vi "Flatten to protobuf.vi"(8 "error in (no error)":errorcluster, 10 "Data":T1) -> (0 "error out":errorcluster, 2 "Buffer":u8[](array[numeric]) format="%.0x")   [LabVIEW 2020, in "PB Msg Template.lvlib"]
uses:
  PB Msg Template.lvlib
  Data.ctl
  LV-Proto/Wire Encode Tag.vi
  LV-Proto/Wire Encode Varint I32.vi
  LV-Proto/LV-Proto.lvlib
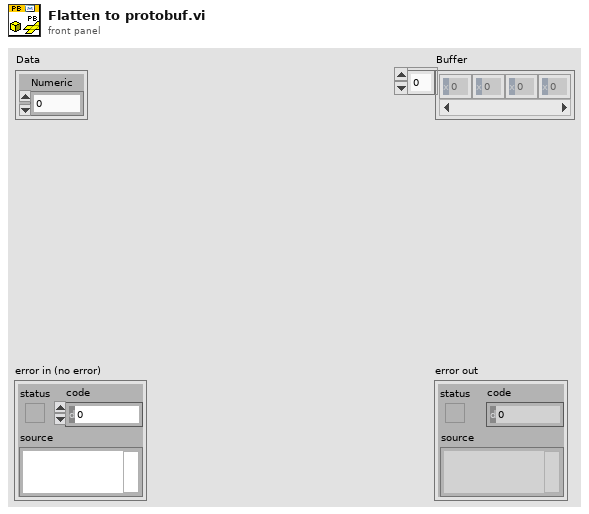
[diagram p1: front panel]
types:
  T1 = typedef "PB Msg Template.lvlib/Data.ctl" = cluster{"Numeric":dbl}
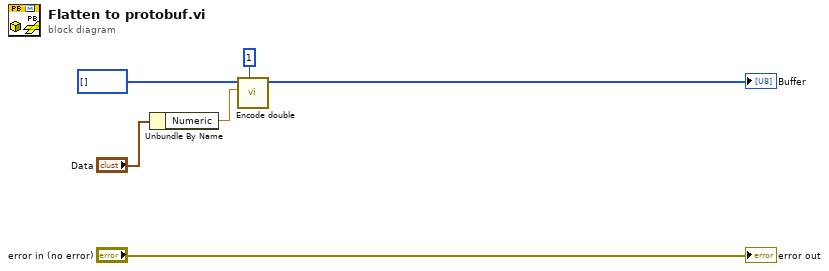
[diagram p0: block diagram]
diagram:
  n1 = Unbundle By Name("Data") -> ("Numeric"=w5:dbl)
  n2 = call "Encode double.vi"("Field Number"=1, "double"=w5, "Buffer in"=u8[] []) -> ("Buffer"=→"Buffer":u8[])  [unwired: 8 in]
  "error out" <- "error in (no error)"
